vi "FB_OP_Lim_knees.vi"(0 "Constants LL":T1, 7 "WirePullComp":bool, 11 "SetTension":dbl[](array[numeric]), 12 "vel (rpm)":dbl[](array[numeric])) -> (15 "PID_OP_Lim":cluster{"PID_OP_upLim":dbl, dbl}[](array[cluster]))   [LabVIEW 2017]
uses:
  typeDef/constants_LL.ctl
  <vilib>/imath/engines/lvmath2/RunTimeEngine/NodeEndStatement/NIMS_NodeEndStatement_Output.vi
  <instcachedir>/0/NIMS_NodeEndStatement_Output_53EC0D466D134D7ABD903AC30B43404B.lvgen/NIMS_NodeEndStatement_Output_53EC0D466D134D7ABD903AC30B43404B_001.vi
  <vilib>/imath/engines/lvmath2/RunTimeEngine/ErrorHandling/NIMS_Finalize Error.vi
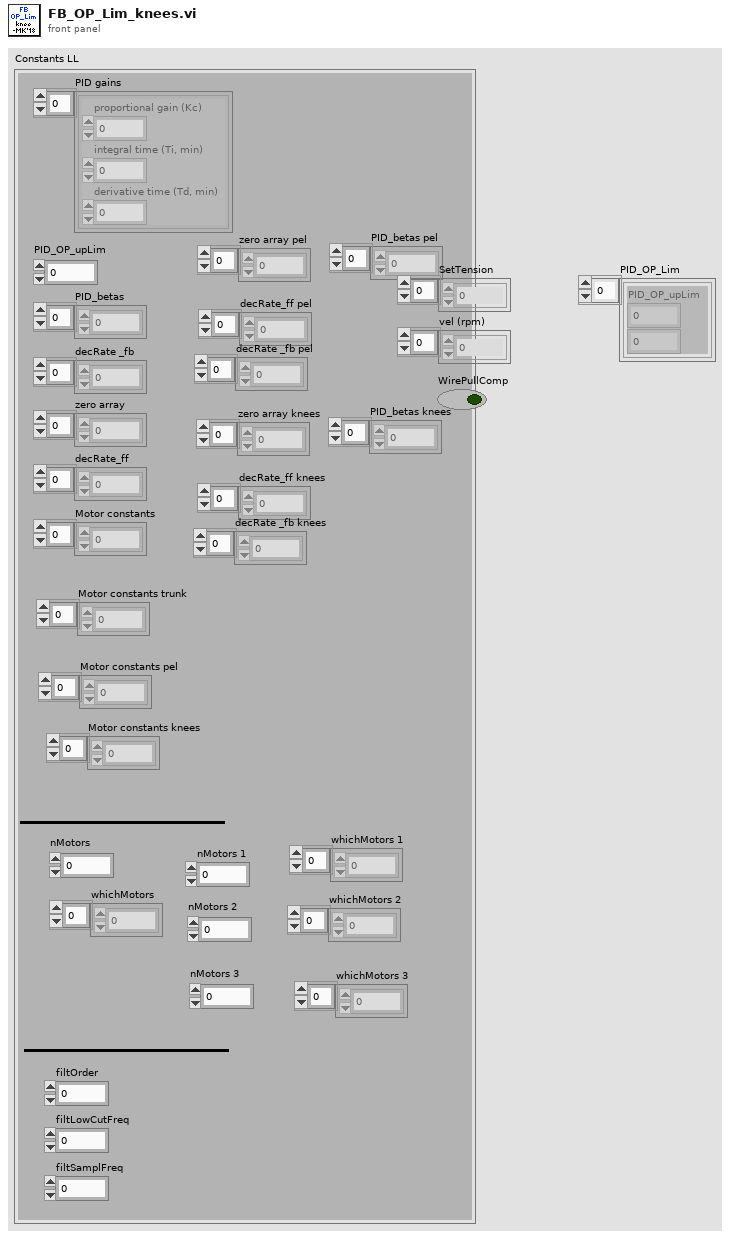
[diagram p1: front panel]
types:
  T1 = typedef "constants_LL.ctl" = cluster{"zero array":dbl[], "decRate_ff":dbl[], "Motor constants":dbl[], "PID gains":cluster{"proportional gain (Kc)":dbl, "integral time (Ti, min)":dbl, "derivative time (Td, min)":dbl}[], "decRate _fb":dbl[], "PID_OP_upLim":dbl, "nMotors":i32, "PID_betas":dbl[], "filtOrder":i32, "filtLowCutFreq":dbl, "filtSamplFreq":dbl, "whichMotors":i32[], "nMotors 1":i32, "nMotors 2":i32, "Motor constants pel":dbl[], "Motor constants trunk":dbl[], "whichMotors 1":i32[], "whichMotors 2":i32[], "zero array pel":dbl[], "decRate_ff pel":dbl[], "decRate _fb pel":dbl[], "PID_betas pel":dbl[], "whichMotors 3":i32[], "nMotors 3":i32, "Motor constants knees":dbl[], "zero array knees":dbl[], "decRate_ff knees":dbl[], "decRate _fb knees":dbl[], "PID_betas knees":dbl[]}
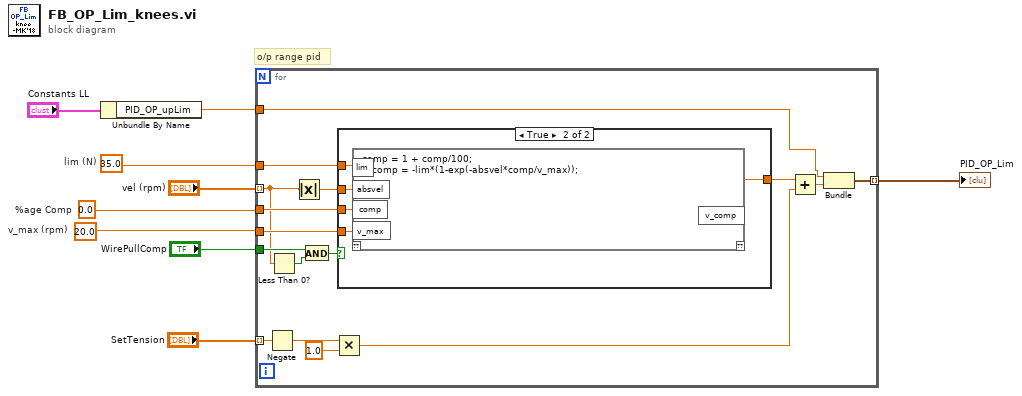
[diagram p0: block diagram]
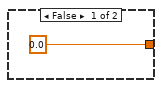
[diagram p2: hidden frame]
diagram:
  w2 = 0.0  # %age Comp
  w3 = 20.0  # v_max (rpm)
  w1 = 35.0  # lim (N)
  # "o/p range pid"
  n1 = Unbundle By Name("Constants LL") -> ("PID_OP_upLim"=w7:dbl)
  n2 = for {
    tunnel: [w25] -> w4 mode=indexing
    tunnel: "vel (rpm)" -> [w12] mode=indexing
    tunnel: "SetTension" -> [w23] mode=indexing
    tunnel: w7 -> [w10]
    tunnel: "WirePullComp" -> [w14]
    tunnel: w2 -> [w19]
    tunnel: w1 -> [w17]
    tunnel: w3 -> [w16]
    n3 = Negate(x=w23) -> (-x=w22:dbl)
    n4 = Less Than 0?(x=w12) -> (x < 0?=w13:bool)
    n5 = Absolute Value(x=w12) -> (abs(x)=w11:dbl)
    n6 = And(x=w14, y=w13) -> (x .and. y?=w15:bool)
    n7 = Multiply(x=w22, y=1.0) -> (x*y=w21:dbl)
    n8 = case shown="True" w15 {
      tunnel: [0.0 ("f") w31] -> w18
      tunnel: w19 -> [_ w30]
      tunnel: w11 -> [_ w29]
      tunnel: w17 -> [_ w28]
      tunnel: w16 -> [_ w27]
      frame False {
      }
      frame True {
        n9 = mathscript code="comp = 1 + comp/100;\nv_comp = -lim*(1-exp(-absvel*comp/v_max));"("lim"=w28, "absvel"=w29, "comp"=w30, "v_max"=w27) -> ("v_comp"=w31:dbl)  [unwired: 1 in, 1 out]
      }
    }
    n10 = Add(x=w18, y=w21) -> (x+y=w24:dbl)
    n11 = Bundle("PID_OP_upLim"=w10, w24) -> (w25:cluster{"PID_OP_upLim":dbl, dbl})  [unwired: 1 in]
  }
  "PID_OP_Lim" <- w4
